vi "Create Tag.vi"(1 "TagY":dbl, 2 "TagX":dbl, 3 "TagID":dbl) -> (0 "Tag Out":refnum<class "Tag.lvclass">)   [LabVIEW 2014, in "Tag.lvclass"]
uses:
  Tag.lvclass
  Tag.lvclass/Tag.ctl
panel:
  in  "PreviousTagY":dbl
  in  "PreviousTagX":dbl
  out "error out":errorcluster
  in  "error in (no error)":errorcluster
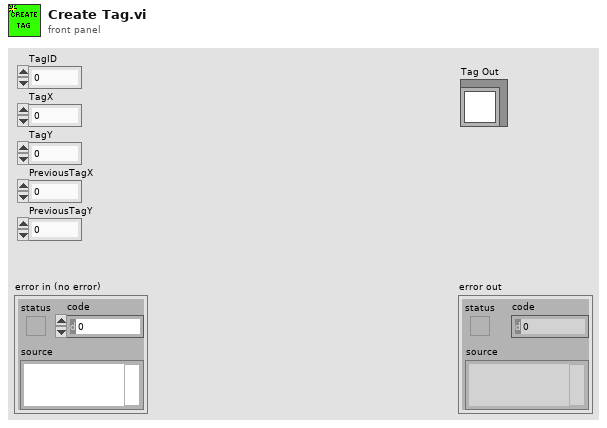
[diagram p1: front panel]
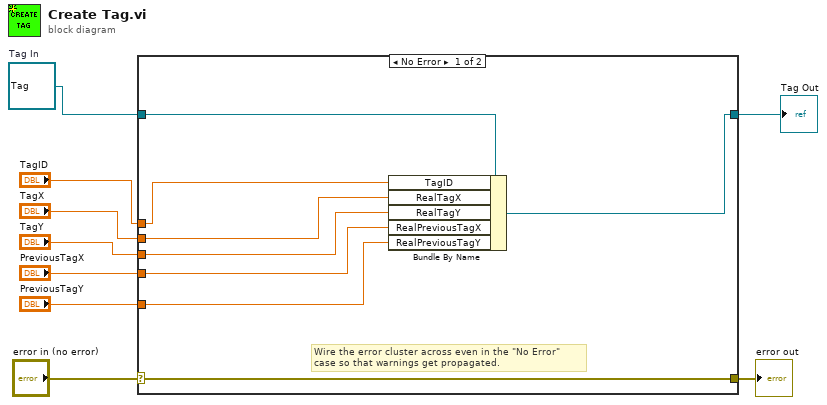
[diagram p0: block diagram]
diagram:
  w4 = refnum<class "Tag.lvclass"> refnum  # Tag In
  n1 = case shown="No Error" "error in (no error)" {
    selector: "error in (no error)" -> [w17 w19]
    tunnel: [w17 w19] -> w8
    tunnel: [w14 w18] -> w3
    tunnel: w4 -> [w15 w18]
    tunnel: "TagID" -> [w16 _]
    tunnel: "TagX" -> [w13 _]
    tunnel: "TagY" -> [w12 _]
    tunnel: "PreviousTagX" -> [w11 _]
    tunnel: "PreviousTagY" -> [w10 _]
    frame No Error {
      # "Wire the error cluster across even in the \"No Error\"\ncase so that warnings get propagated."
      n2 = Bundle By Name(cluster=w15, "TagID"=w16, "RealTagX"=w13, "RealTagY"=w12, "RealPreviousTagX"=w11, "RealPreviousTagY"=w10) -> (w14:refnum<class "Tag.lvclass">)
    }
    frame Error {
    }
  }
  "error out" <- w8
  "Tag Out" <- w3
